vi "Checksum Pass.vi"(4 "Message In":string) -> (1 "Checksum Pass":bool)   [LabVIEW 2012, in "MicroStrain 3DM-GXx.lvlib"]
doc: "Takes a complete message and returns the result of the checksum test. True indicates a valid message, false indicates an invalid message."
uses:
  <instrlib>/MicroStrain 3DM-GXx/MicroStrain 3DM-GXx.lvlib
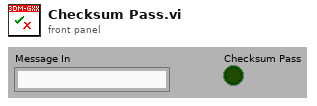
[diagram p1: front panel]
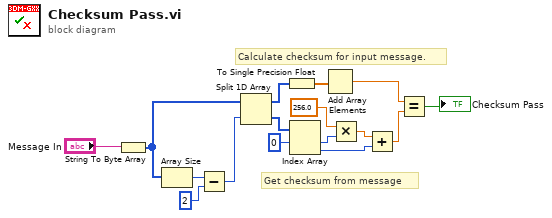
[diagram p0: block diagram]
diagram:
  # "Calculate checksum for input message."
  # "Get checksum from message"
  n1 = String To Byte Array(string="Message In") -> (unsigned byte array=w5:u8[])
  n2 = Array Size(array=w5) -> (size(s)=w16:i32)
  n3 = Subtract(x=w16, y=2) -> (x-y=w14:i32)
  n4 = Split 1D Array(array=w5, index=w14) -> (first subarray=w3:u8[], second subarray=w13:u8[])
  n5 = To Single Precision Float(number=w3) -> (single precision float=w2:sgl[])
  n6 = Index Array(array=w13, index #1=0 ("index")) -> (element #1=w10:u8, element #2=w8:u8)  [unwired: 1 in]
  n7 = Add Array Elements(numeric array=w2) -> (sum=w1:sgl)
  n8 = Multiply(x=256.0, y=w10) -> (x*y=w9:dbl)
  n9 = Add(x=w9, y=w8) -> (x+y=w7:dbl)
  n10 = Equal?(x=w1, y=w7) -> (x = y?=→"Checksum Pass":bool)
